vi "Release Priority Queue.vi"(8 "error in (no error)":errorcluster, 9 "force destroy? (F)":bool, 11 "Priority Queue":refnum<class "Priority Queue.lvclass">) -> (0 "error out":errorcluster)   [LabVIEW 2020, in "Communicable State Machine.lvlib" / "Priority Queue.lvclass"]
uses:
  Priority Queue.lvclass
  Priority Queue.lvclass/Priority Queue.ctl
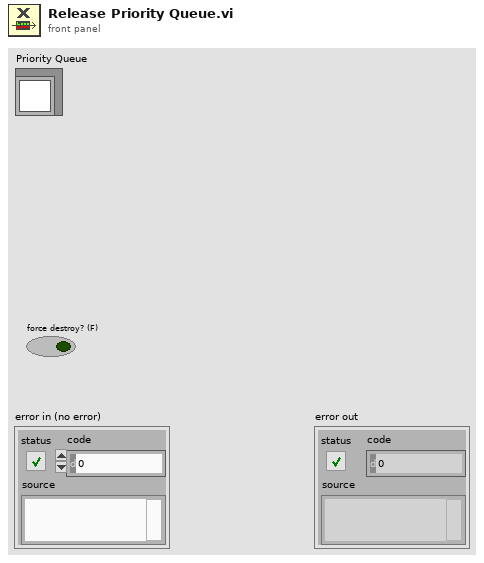
[diagram p1: front panel]
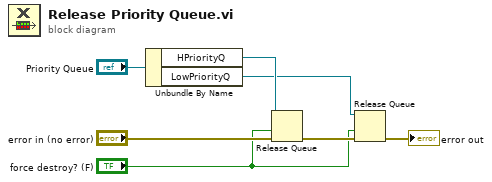
[diagram p0: block diagram]
diagram:
  n1 = Unbundle By Name("Priority Queue") -> ("HPriorityQ"=w6:refnum<queue>, "LowPriorityQ"=w5:refnum<queue>)
  n2 = Release Queue(queue=w6, force destroy? (F)="force destroy? (F)", error in (no error)="error in (no error)") -> (error out=w3:errorcluster)  [unwired: 2 out]
  n3 = Release Queue(queue=w5, force destroy? (F)="force destroy? (F)", error in (no error)=w3) -> (error out=→"error out":errorcluster)  [unwired: 2 out]
